vi "Initialize.vi"(8 "Error In":errorcluster) -> (0 "Error Out":errorcluster, 3 "Queue out":refnum<queue>)   [LabVIEW 2019, in "Controller.lvlib"]
uses:
  Controller.lvlib
  Queues/Message Cluster.ctl
  Queues/Queues.lvlib
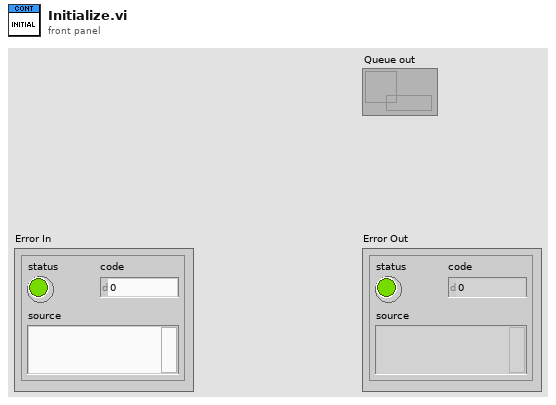
[diagram p1: front panel]
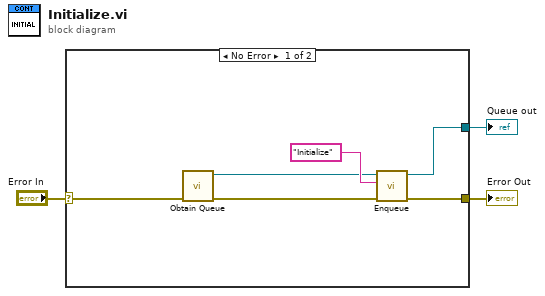
[diagram p0: block diagram]
diagram:
  n1 = case shown="No Error" "Error In" {
    selector: "Error In" -> [w6 w10]
    tunnel: [w8 w10] -> w3
    tunnel: [w4 _] -> w1
    frame No Error {
      n2 = call "Obtain Queue.vi"("Error In"=w6) -> ("Error Out"=w5:errorcluster, "Queue out"=w7:refnum<queue>)  [unwired: 9 in]
      n3 = call "Enqueue.vi"("Error In"=w5, "State"="Initialize", "Queue in"=w7) -> ("Error Out"=w8:errorcluster, "Queue out"=w4:refnum<queue>)  [unwired: 7 in]
    }
    frame Error {
    }
  }
  "Error Out" <- w3
  "Queue out" <- w1
